vi "Disable motor.vi"   [LabVIEW 2010]
panel:
  # "disables motor"
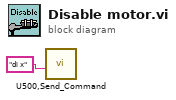
[diagram p0: block diagram]
diagram:
  n1 = call "U500,Send_Command.vi"("Command String"="di x") -> ()  [unwired: 9 in, 2 out]
